vi "Config Program Type vi.vi"(8 "error in (no error)":errorcluster, 11 "SEQ":refnum<queue>) -> (0 "error out":errorcluster, 1 "Program Type":string, 3 "SEQ Out":refnum<queue>)   [LabVIEW 2014, in "SeqLoop.lvlib"]
uses:
  SeqLoop.lvlib
  APIs/Message Queue/Message Cluster.ctl
  APIs/Message Queue/WINFAS 2 Message Queue.lvlib
panel:
  in  "Scale":bool
  in  "Tapons":bool
  in  "Close":bool
  in  "Cap":bool
  in  "Engranometer":bool
  # "Seleccione el tipo de maquina que desea usar para el programa configurado."
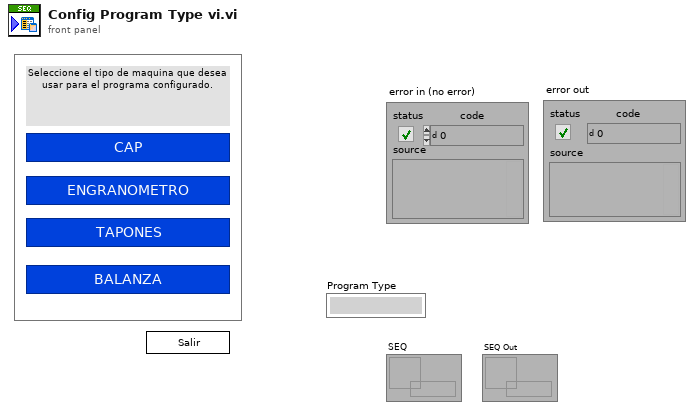
[diagram p1: front panel]
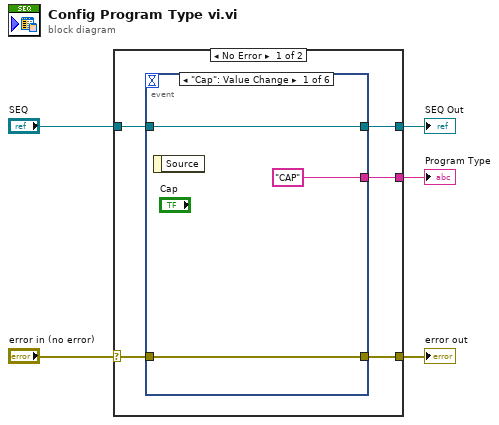
[diagram p0: block diagram]
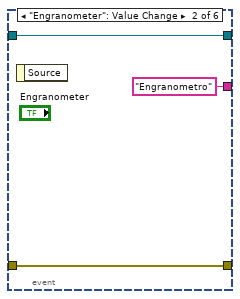
[diagram p2: hidden frame]
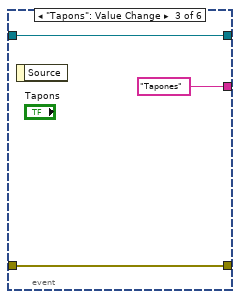
[diagram p3: hidden frame]
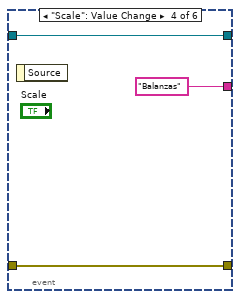
[diagram p4: hidden frame]
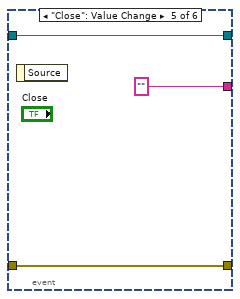
[diagram p5: hidden frame]
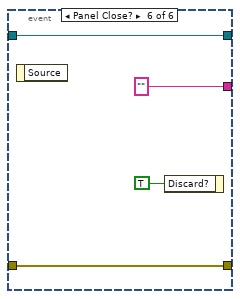
[diagram p6: hidden frame]
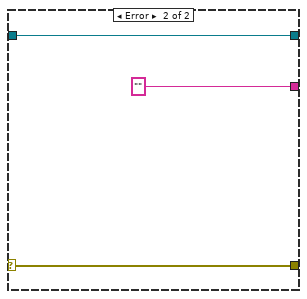
[diagram p7: hidden frame]
diagram:
  n1 = case shown="No Error" "error in (no error)" {
    selector: "error in (no error)" -> [w10 w32]
    tunnel: [w9 w32] -> w4
    tunnel: [w8 ""] -> w3
    tunnel: [w7 w30] -> w2
    tunnel: "SEQ" -> [w6 w30]
    frame No Error {
      n2 = event shown="[0] \"Cap\": Value Change" {
        selector: _ -> [_ _ _ _ _ _]
        dyn-events: _ -> [_ _ _ _ _ _]
        timeout: _ -> [_ _ _ _ _ _]
        tunnel: w10 -> [w13 w16 w19 w21 w25 w28]
        tunnel: [w13 w16 w19 w21 w25 w28] -> w9
        tunnel: ["CAP" "Engranometro" "Tapones" "Balanzas" "" ""] -> w8
        tunnel: [w11 w14 w17 w20 w23 w26] -> w7
        tunnel: w6 -> [w11 w14 w17 w20 w23 w26]
        event "Cap": Value Change {
          n3 = event-data() -> ()  [unwired: 1 in, 1 out]
        }
        event "Engranometer": Value Change {
          n4 = event-data() -> ()  [unwired: 1 in, 1 out]
        }
        event "Tapons": Value Change {
          n5 = event-data() -> ()  [unwired: 1 in, 1 out]
        }
        event "Scale": Value Change {
          n6 = event-data() -> ()  [unwired: 1 in, 1 out]
        }
        event "Close": Value Change {
          n7 = event-data() -> ()  [unwired: 1 in, 1 out]
        }
        event Panel Close? {
          n8 = event-data() -> ()  [unwired: 1 in, 1 out]
          n9 = event-data("Discard?"=TRUE) -> ()  [unwired: 1 in, 1 out]
        }
      }
    }
    frame Error {
    }
  }
  "error out" <- w4
  "Program Type" <- w3
  "SEQ Out" <- w2
